vi "readFromXML.vi"(8 "error in (no error)":errorcluster, 10 "XMLin":string, 11 "TCSTcsCommand in":refnum<class "TCSTcsCommand.lvclass">) -> (0 "error out":errorcluster, 3 "TCSTcsCommand out":refnum<class "TCSTcsCommand.lvclass">)   [LabVIEW 2022 SP3, in "TCSDataDefinitions.lvlib" / "TCSCommand.lvlib" / "TCSTcsCommand.lvclass"]
uses:
  TCSTcsCommand.lvclass
  TCSCommand/TCSCommand.lvclass
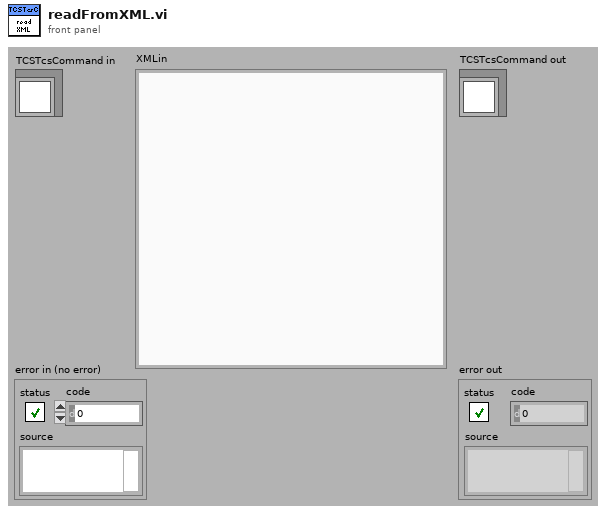
[diagram p1: front panel]
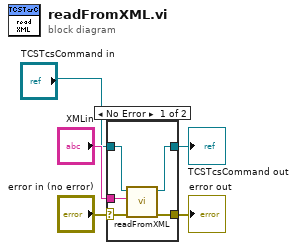
[diagram p0: block diagram]
diagram:
  n1 = case shown="No Error" "error in (no error)" {
    selector: "error in (no error)" -> [w7 w12]
    tunnel: [w8 w12] -> w4
    tunnel: [w9 w11] -> w3
    tunnel: "TCSTcsCommand in" -> [w10 w11]
    tunnel: "XMLin" -> [w6 _]
    frame No Error {
      n2 = call-parent "readFromXML.vi"("error in (no error)"=w7, "XML in"=w6, "TCSCommand in"=w10) -> ("error out"=w8:errorcluster, "TCSCommand out"=w9:refnum<class "TCSTcsCommand.lvclass">)  [unwired: 7 in]
    }
    frame Error {
    }
  }
  "error out" <- w4
  "TCSTcsCommand out" <- w3
